vi "test21-LosslessRegisterStateMultipleTimesNonCSM.vi"(8 "error in (no error)":errorcluster, 11 "TestCase in":refnum<class "testcase-CSMBroadcast.lvclass">) -> (0 "error out":errorcluster, 3 "TestCase out":refnum<class "testcase-CSMBroadcast.lvclass">)   [LabVIEW 2017, in "testcase-CSMBroadcast.lvclass"]
uses:
  testcase-CSMBroadcast.lvclass
  <vilib>/addons/_JKI Toolkits/VI Tester/TestCase.llb/TestCase.lvclass
  src/user.lib/_NEVSTOP/Communicable State Machine(CSM)/Communicable State Machine.lvlib
  CSM/CSM-Testcase.lvlib
  C:/Program Files (x86)/National Instruments/LabVIEW 2017/vi.lib/addons/_JKI Toolkits/VI Tester/TestCase.llb/TestCase.lvclass
panel:
  out "Arguments":string
  out "ModuleName":string
  out "LoopCount":i32
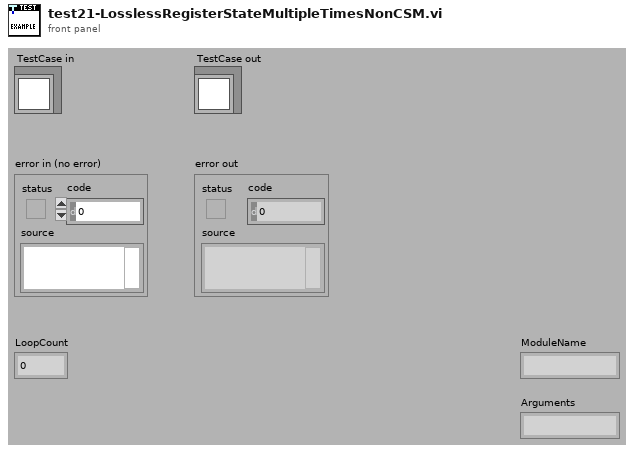
[diagram p1: front panel]
types:
  T1 = cluster{"ModuleName":string, "Status":string, "Arguments":string}
  T2 = cluster{"cluster":cluster{"ModuleName":string, "Status":string, "Arguments":string}, "Counter":u32}
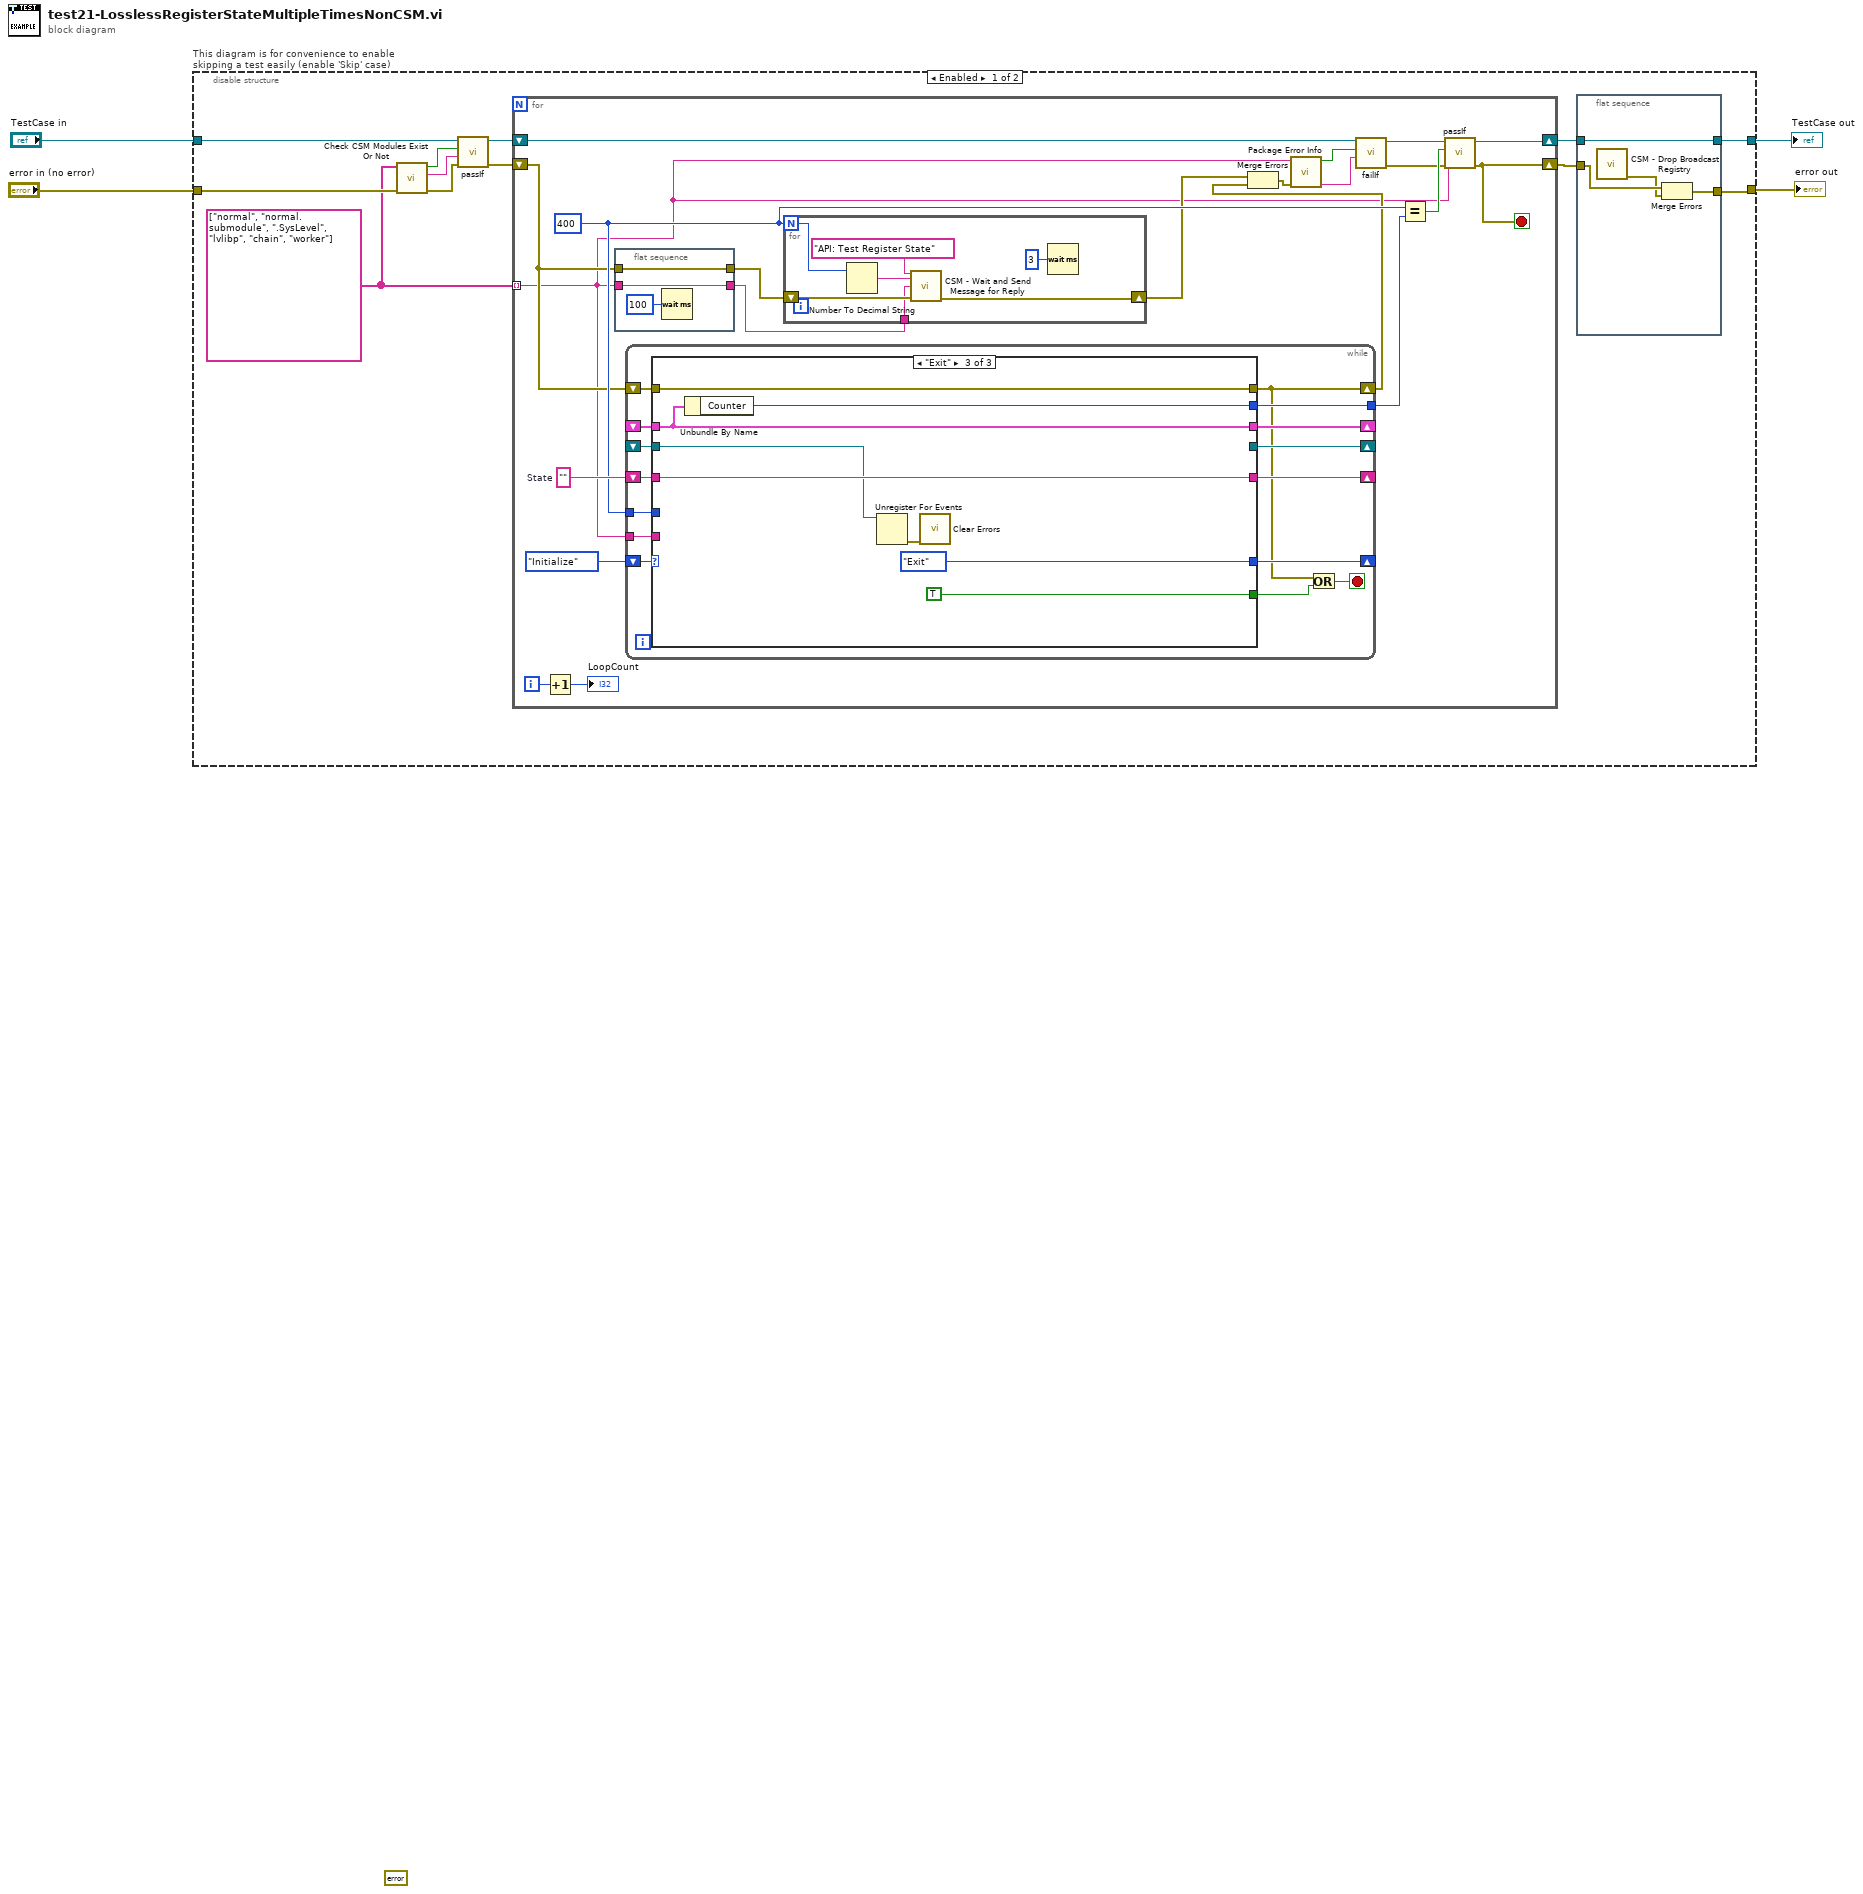
[diagram p0: block diagram]
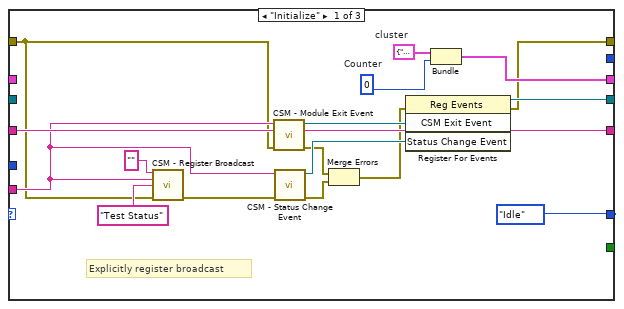
[diagram p2: hidden frame]
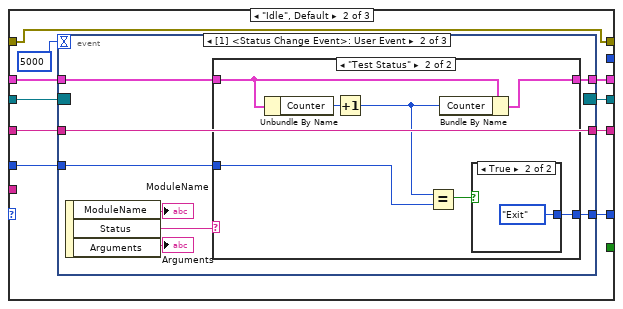
[diagram p3: hidden frame]
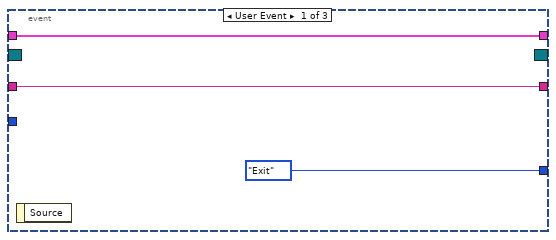
[diagram p4: hidden frame]
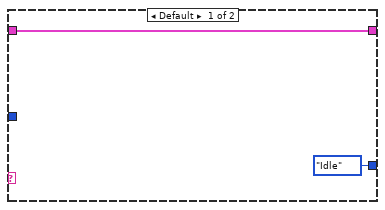
[diagram p5: hidden frame]
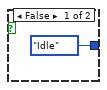
[diagram p6: hidden frame]
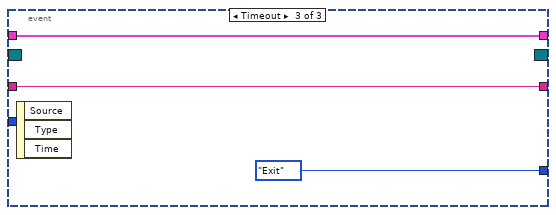
[diagram p7: hidden frame]
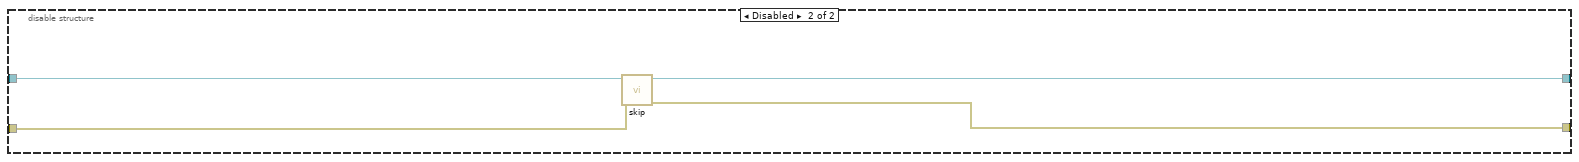
[diagram p8: hidden frame]
diagram:
  (unwired) errorcluster {"status"=FALSE, "code"=0, "source"=""} ("error out")
  n1 = disable-structure "This diagram is for convenience to enable skipping a test easily (enable 'Skip' case)" shown="Enabled" {
    disable-tunnel: "TestCase in" -> [w11 w130]
    disable-tunnel: [w5 w128] -> w2
    disable-tunnel: [w15 w129] -> w1
    disable-tunnel: "error in (no error)" -> [w8 w127]
    frame Enabled {
      w7 = string[] ["normal", "normal.submodule", ".SysLevel", "lvlibp", "chain", "worker"]
      n2 = call "Check CSM Modules Exist Or Not.vi"("error in"=w8, "CSM names in"=w7) -> ("error out"=w12:errorcluster, "Debug string"=w13:string, "All Modules Exist?"=w14:bool)  [unwired: 7 in]
      n3 = call-dynamic "passIf.vi"("error in (no error)"=w12, "message (\"\")"=w13, "pass"=w14, "TestCase in"=w11) -> ("error out"=w9:errorcluster, "TestCase out"=w10:refnum<class "testcase-CSMBroadcast.lvclass">)  [unwired: 6 in]
      n4 = for {
        shift-right: [w39] -> w6
        shift-left: w10 -> [w23]
        shift-right: [w36] -> w16
        shift-left: w9 -> [w30]
        tunnel: w7 -> [w24] mode=indexing
        i -> [w38]
        stop <- w36 stop-if-true
        w32 = 400
        w40 = ""  # State
        n5 = Increment(x=w38) -> (x+1=→"LoopCount":i32)
        n6 = flat-sequence {
          tunnel: w24 -> [w51]
          tunnel: [w51] -> w35
          tunnel: w30 -> [w49]
          tunnel: [w49] -> w31
          frame #0 {
            n7 = Wait (ms)(milliseconds to wait=u32 100) -> ()  [unwired: 1 out]
          }
        }
        n8 = while {
          shift-right: [w65] -> _
          shift-left: enum16{"Idle", "Initialize", "Exit"}."Initialize" -> [w66]
          shift-right: [w63] -> _
          shift-left: w40 -> [w64]
          shift-right: [w62] -> _
          shift-left: _ -> [w61]
          shift-right: [w60] -> _
          shift-left: _ -> [w59]
          tunnel: w24 -> [w58]
          tunnel: [w57] -> w34
          tunnel: w32 -> [w56]
          shift-right: [w54] -> w27
          shift-left: w30 -> [w55]
          stop <- w52 stop-if-true
          n9 = case shown="\"Exit\"" w66 {
            tunnel: [enum16{"Idle", "Initialize", "Exit"}."Idle" w93 enum16{"Idle", "Initialize", "Exit"}."Exit"] -> w65
            tunnel: [_ _ TRUE] -> w53
            tunnel: w64 -> [w82 w91 w124]
            tunnel: [w82 w92 w124] -> w63
            tunnel: [w80 w89 _] -> w62
            tunnel: w61 -> [_ w90 w123]
            tunnel: [w79 w87 w120] -> w60
            tunnel: w59 -> [_ w88 w120]
            tunnel: w58 -> [w71 _ _]
            tunnel: [_ _ w121] -> w57
            tunnel: w56 -> [_ w85 _]
            tunnel: w55 -> [w69 w84 w119]
            tunnel: [w67 w84 w119] -> w54
            frame "Initialize" {
              w74 = u32 0  # Counter
              w77 = T1 {"ModuleName"="", "Status"="", "Arguments"=""}  # cluster
              # "Explicitly register broadcast"
              n10 = call "CSM - Register Broadcast.vi"("CSM Name(Empty for Broadcast Event)"="", "Source CSM Name (* as Default)"=w71, "Trigger"="Test Status" ("State"), "Error In"=w69) -> ("error out"=w70:errorcluster)  [unwired: 10 in, 1 out]
              n11 = call "CSM - Module Exit Event.vi"("Error In"=w69, "Name (\"\" to Use UUID) In"=w71) -> ("error out"=w76:errorcluster, "CSM Exit Event"=w81:refnum<user-event>)  [unwired: 7 in, 1 out]
              n12 = call "CSM - Status Change Event.vi"("Error In"=w70, "CSM Module"=w71) -> ("error out"=w75:errorcluster, "Status Change Event"=w78:refnum<user-event>)  [unwired: 7 in, 1 out]
              n13 = Merge Errors(w76, w75) -> (w68:errorcluster)
              n14 = register-events(error in=w68, w81, w78) -> (reference out=w80:refnum<event-registration>, error out=w67:errorcluster)  [unwired: 1 in]
              n15 = Bundle("cluster"=w77, "Counter"=w74) -> (w79:T2)  [unwired: 1 in]
            }
            frame "Idle", Default {
              n16 = event shown="[1] <Status Change Event>: User Event" {
                selector: w90 -> [_ _ _]
                dyn-events: [_ _ _] -> w89
                timeout: 5000 -> [_ _ _]
                tunnel: [enum16{"Idle", "Initialize", "Exit"}."Exit" w103 enum16{"Idle", "Initialize", "Exit"}."Exit"] -> w93
                tunnel: w91 -> [w96 w104 w118]
                tunnel: [w96 w104 w118] -> w92
                tunnel: w88 -> [w94 w101 w117]
                tunnel: [w94 w102 w117] -> w87
                tunnel: w85 -> [_ w100 _]
                event User Event {
                  n17 = event-data() -> ()  [unwired: 1 in, 1 out]
                }
                event User Event {
                  n18 = event-data() -> ("ModuleName"=→"ModuleName":string, "Status"=w99:string, "Arguments"=→"Arguments":string)  [unwired: 1 in]
                  n19 = case shown="\"Test Status\"" w99 {
                    tunnel: [enum16{"Idle", "Initialize", "Exit"}."Idle" w113] -> w103
                    tunnel: [w106 w112] -> w102
                    tunnel: w101 -> [w106 w111]
                    tunnel: w100 -> [_ w107]
                    frame Default {
                    }
                    frame "Test Status" {
                      n20 = Unbundle By Name(w111) -> ("Counter"=w110:u32)
                      n21 = Increment(x=w110) -> (x+1=w108:u32)
                      n22 = Equal?(x=w108, y=w107) -> (x = y?=w109:bool)
                      n23 = Bundle By Name(cluster=w111, "Counter"=w108) -> (w112:T2)
                      n24 = case shown="True" w109 {
                        tunnel: [enum16{"Idle", "Initialize", "Exit"}."Idle" enum16{"Idle", "Initialize", "Exit"}."Exit"] -> w113
                        frame False {
                        }
                        frame True {
                        }
                      }
                    }
                  }
                }
                event Timeout {
                  n25 = event-data() -> ()  [unwired: 1 in, 3 out]
                }
              }
            }
            frame "Exit" {
              n26 = Unbundle By Name(w120) -> ("Counter"=w121:u32)
              n27 = Unregister For Events(event registration refnum=w123) -> (error out=w122:errorcluster)  [unwired: 1 in]
              n28 = call <vilib>:"Clear Errors.vi"("error in (no error)"=w122) -> ()  [unwired: 5 in, 2 out]
            }
          }
          n29 = Or(x=w54, y=w53) -> (x .or. y?=w52:bool)
        }
        n30 = for {
          N: w32 -> [w46]
          shift-right: [w44] -> w25
          shift-left: w31 -> [w45]
          tunnel: w35 -> [w43]
          n31 = Number To Decimal String(number=w46) -> (decimal integer string=w47:string)  [unwired: 1 in]
          n32 = call "CSM - Wait and Send Message for Reply.vi"("State"="API: Test Register State", "Arguments (\"\")"=w47, "Target Module"=w43, "Error In (No Error)"=w45) -> ("error out"=w44:errorcluster)  [unwired: 8 in, 3 out]
          n33 = Wait (ms)(milliseconds to wait=u32 3) -> ()  [unwired: 1 out]
        }
        n34 = Merge Errors(w25, w27) -> (w26:errorcluster)
        n35 = call "Package Error Info.vi"("error in"=w26, "String in"=w24) -> ("packed error info out"=w28:string, "error status"=w29:bool)  [unwired: 8 in]
        n36 = call-dynamic "failIf.vi"("message (\"\")"=w28, "fail"=w29, "TestCase in"=w23) -> ("error out"=w21:errorcluster, "TestCase out"=w22:refnum<class "testcase-CSMBroadcast.lvclass">)  [unwired: 7 in]
        n37 = Equal?(x=w32, y=w34) -> (x = y?=w33:bool)
        n38 = call-dynamic "passIf.vi"("error in (no error)"=w21, "message (\"\")"=w24, "pass"=w33, "TestCase in"=w22) -> ("error out"=w36:errorcluster, "TestCase out"=w39:refnum<class "testcase-CSMBroadcast.lvclass">)  [unwired: 6 in]
      }
      n39 = flat-sequence {
        tunnel: w16 -> [w20]
        tunnel: [w19] -> w15
        tunnel: w6 -> [w17]
        tunnel: [w17] -> w5
        frame #0 {
          n40 = call "CSM - Drop Broadcast Registry.vi"() -> ("error out"=w18:errorcluster)  [unwired: 15 in]
          n41 = Merge Errors(w20, w18) -> (w19:errorcluster)
        }
      }
    }
    frame Disabled {
      # "skip test result while test is under development"
      n42 = call <vilib>:"skip.vi"("error in (no error)"=w127, "TestCase in"=w130) -> ("error out"=w129:errorcluster, "TestCase out"=w128:refnum<class "testcase-CSMBroadcast.lvclass">)  [unwired: 8 in]
    }
  }
  "error out" <- w1
  "TestCase out" <- w2
